vi "zadanie_2.vi"() -> ()   [LabVIEW 2020]
panel:
  out "trimmed string":string
  in  "stop":bool
  in  "wejscie":string
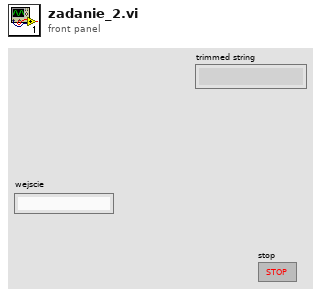
[diagram p1: front panel]
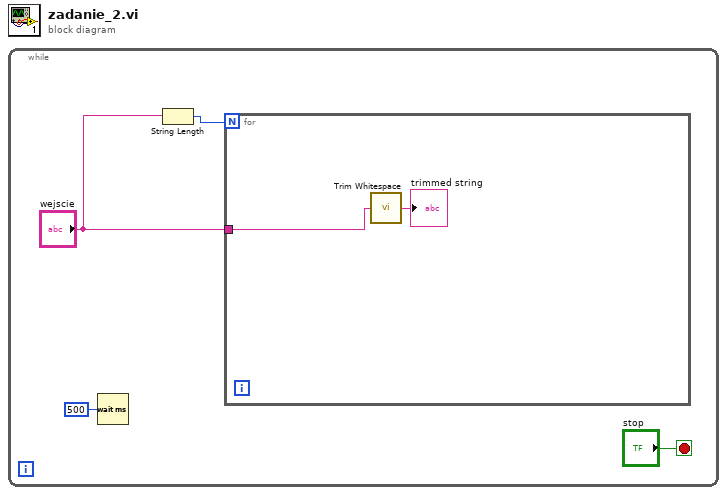
[diagram p0: block diagram]
diagram:
  n1 = while {
    stop <- "stop" stop-if-true
    n2 = Wait (ms)(milliseconds to wait=u32 500) -> ()  [unwired: 1 out]
    n3 = String Length(string="wejscie") -> (length=w4:i32)
    n4 = for {
      N: w4 -> [_]
      tunnel: "wejscie" -> [w6]
      n5 = call <vilib>:"Trim Whitespace.vi"("string"=w6) -> ("trimmed string"=→"trimmed string":string)  [unwired: 1 in]
    }
  }
